vi "Write Linked List Ref .vi"(8 "error in (no error)":errorcluster, 10 "Linked List Ref":refnum<data-value>, 11 "User Configuration Manager in":refnum<class "User Configuration Manager.lvclass">) -> (0 "error out":errorcluster, 3 "User Configuration Manager out":refnum<class "User Configuration Manager.lvclass">)   [LabVIEW 2017, in "User Configuration Manager.lvlib" / "User Configuration Manager.lvclass"]
uses:
  User Configuration Manager.lvclass
  <vilib>/gpm_packages/@cs/linked-list/Source/Linked List/ILinkedList/ILinked List.lvclass
  User Configuration Manager.lvclass/User Configuration Manager.ctl
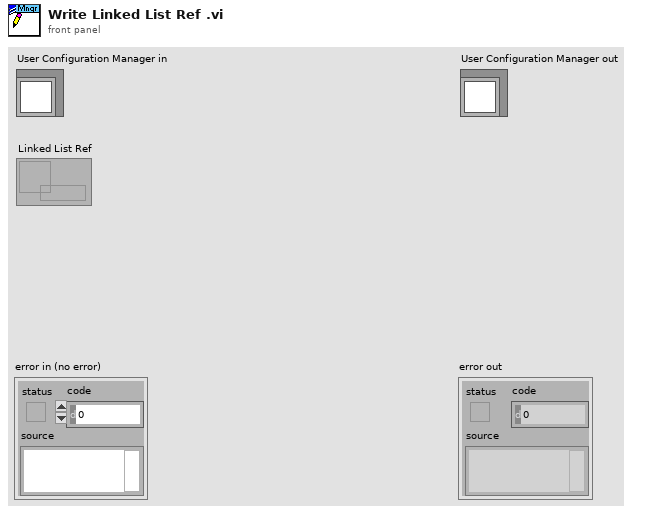
[diagram p1: front panel]
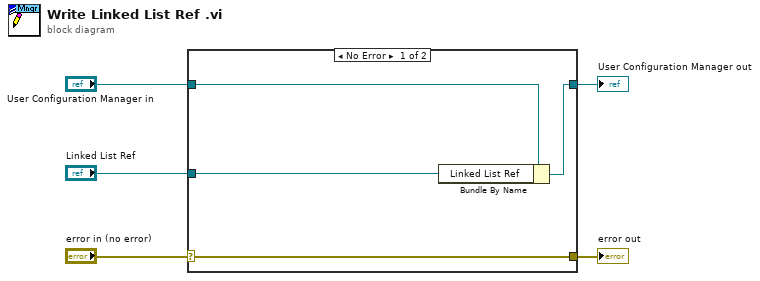
[diagram p0: block diagram]
diagram:
  n1 = case shown="No Error" "error in (no error)" {
    selector: "error in (no error)" -> [w9 w10]
    tunnel: [w9 w10] -> w4
    tunnel: [w7 w11] -> w2
    tunnel: "User Configuration Manager in" -> [w8 w11]
    tunnel: "Linked List Ref" -> [w6 _]
    frame No Error {
      n2 = Bundle By Name(cluster=w8, "Linked List Ref"=w6) -> (w7:refnum<class "User Configuration Manager.lvclass">)
    }
    frame Error {
    }
  }
  "error out" <- w4
  "User Configuration Manager out" <- w2
